vi "Set BD string constant value.vi"(8 "error in (no error)":errorcluster, 9 "Name of string constant":string="CD_CHM_FileName", 10 "New String Value":string, 11 "Path to VI":path) -> (0 "error out":errorcluster)   [LabVIEW 2015, in "NIVS_Consolidated_CDW_MetaDataObj.lvclass"]
doc: "This VI allows you to set the value of a string constant on the target block diagram by name."
uses:
  NIVS_Consolidated_CDW_MetaDataObj.lvclass
  <vilib>/Utility/traverseref.llb/TRef TravTarget.ctl
  <vilib>/Utility/traverseref.llb/VI Scripting - Traverse.lvlib
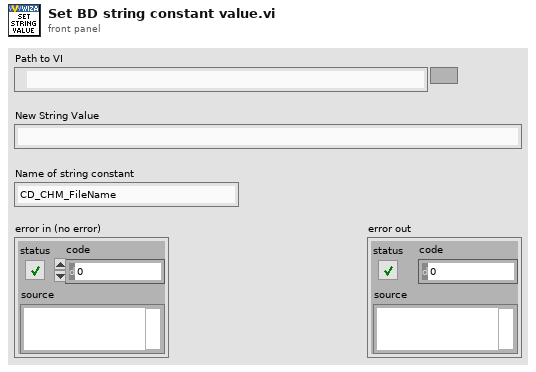
[diagram p1: front panel]
types:
  T1 = typedef "TRef TravTarget.ctl" = enum16{"FP", "BD", "Other"}
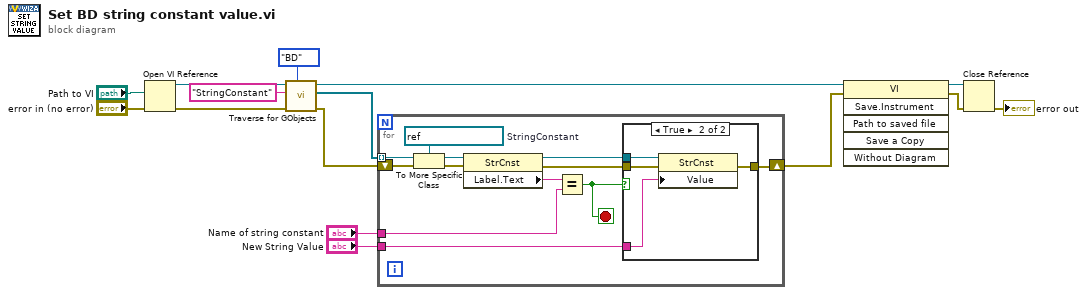
[diagram p0: block diagram]
diagram:
  n1 = Open VI Reference(vi path="Path to VI", error in (no error)="error in (no error)") -> (vi reference=w7:refnum<vi>, error out=w8:errorcluster)  [unwired: 4 in]
  n2 = call <vilib>:"Traverse for GObjects.vi"("Traverse Target"=TRef_TravTarget."BD", "error in (no error)"=w8, "Class Name"="StringConstant", "VI Refnum"=w7) -> ("error out"=w3:errorcluster, "References"=w2:refnum<vi>[], "dup VI Refnum"=w9:refnum<vi>)  [unwired: 4 in, 1 out]
  n3 = for {
    tunnel: w2 -> [w27] mode=indexing
    shift-right: [w17] -> w13
    shift-left: w3 -> [w25]
    tunnel: "Name of string constant" -> [w21]
    tunnel: "New String Value" -> [w18]
    stop <- w16 stop-if-true
    w26 = refnum<vi> refnum  # StringConstant
    n4 = To More Specific Class(target class=w26, reference=w27, error in=w25) -> (specific class reference=w24:refnum<vi>, error out=w23:errorcluster)
    n5 = property class="StrCnst"(reference=w24, error in=w23) -> (reference out=w20:refnum<vi>, error out=w19:errorcluster, "Label.Text"=w22:string)
    n6 = Equal?(x=w22, y=w21) -> (x = y?=w16:bool)
    n7 = case shown="True" w16 {
      tunnel: w20 -> [_ w31]
      tunnel: w19 -> [w28 w29]
      tunnel: w18 -> [_ w30]
      tunnel: [w28 w32] -> w17
      frame False {
      }
      frame True {
        n8 = property class="StrCnst"(reference=w31, error in=w29, "Value"=w30) -> (error out=w32:errorcluster)  [unwired: 1 out]
      }
    }
  }
  n9 = invoke class="VI" method="Save.Instrument"(reference=w9, error in=w13) -> (reference out=w10:refnum<vi>, error out=w11:errorcluster)  [unwired: 4 in, 4 out]
  n10 = Close Reference(reference=w10, error in (no error)=w11) -> (error out=→"error out":errorcluster)
